vi "XY Scanning with Alazar.vi"() -> ()   [LabVIEW 2018]
uses:
  General/Controls/System Parameters.ctl
  General/Controls/Optical Parameters.ctl
  General/Controls/Vibratome Parameters.ctl
  General/Controls/Translation Stage Parameters.ctl
  Hardware Mfg/Thorlabs Translation Stages/Controls/Translation Stage Cluster.ctl
  General/Controls/Translation Stage Types.ctl
  General/Controls/Imaging Parameters.ctl
  General/Controls/Scan Direction.ctl
  Hardware Mfg/AlazarTech SDK/Controls/Clock Controls.ctl
  Hardware Mfg/AlazarTech SDK/Controls/Alazar Device ID.ctl
  Hardware Mfg/AlazarTech SDK/Controls/Channel Input Controls.ctl
  Hardware Mfg/AlazarTech SDK/Controls/General Trigger Settings.ctl
  Hardware Mfg/AlazarTech SDK/Controls/Trigger Engine Controls.ctl
  Hardware Mfg/AlazarTech SDK/Controls/Alazar Acquisition Settings.ctl
  Hardware Mfg/AlazarTech SDK/Controls/Alazar Engine Actions.ctl
  <vilib>/ErrorRing/Error Ring.xnode
panel:
  out "error out":errorcluster
  in  "stop":bool
  in  "Acq Settings":T1={"Window Type"=1, "Record Length"=1536, "Footer"=0, "Output Format"=11, "Offset"=0, "Records Per Buffer"=1000, "Records Count (Records/Acq)"=2147483647} {"Window Type" items=["DSP_WINDOW_NONE", "DSP_WINDOW_HANNING", "DSP_WINDOW_HAMMING", "DSP_WINDOW_BLACKMAN", "DSP_WINDOW_BLACKMAN_HARRIS", "DSP_WINDOW_BARTLETT"]; "Footer" items=["FOOTER_NONE", "FOOTER_NPT"]; "Output Format" items=["FLOAT_AMP2"=10, "FLOAT_LOG"=11]}
  in  "Trigger Settings":T4={"General Trigger Settings"={"Trigger Operation"=0, "Coupling ID"=2, "Range ID"=0, "Delay"=0, "Timeout Ticks"=0, "Mode"=0, "Parameter"=0}, "Trigger Engine 1"={"Trigger Engine"=0, "Source"=0, "Slope"=1, "Level"=0}, "Trigger Engine 2"={"Trigger Engine"=0, "Source"=0, "Slope"=1, "Level"=0}} {"General Trigger Settings"."Trigger Operation" items=["J", "K", "J OR K", "J AND K", "J XOR K", "J AND NOT K", "NOT J AND K"]; "General Trigger Settings"."Coupling ID" items=["AC"=1, "DC"=2]; "General Trigger Settings"."Range ID" items=["5 V", "1 V", "TTL"]; "Trigger Engine 1"."Trigger Engine" items=["J", "K"]; "Trigger Engine 1"."Source" items=["A", "B", "External", "Disable", "C", "D"]; "Trigger Engine 1"."Slope" items=["Positive"=1, "Negative"=2]; "Trigger Engine 2"."Trigger Engine" items=["J", "K"]; "Trigger Engine 2"."Source" items=["A", "B", "External", "Disable", "C", "D"]; "Trigger Engine 2"."Slope" items=["Positive"=1, "Negative"=2]}
  in  "Ch B Input Control":T5={"Channel"=1, "Coupling"=2, "Range"=10, "Impedance"=2} {"Channel" items=["A"=1, "B"=2, "C"=4, "D"=8]; "Coupling" items=["AC"=1, "DC"=2]; "Range" items=["20 mV"=1, "40 mV"=2, "50 mV"=3, "80 mV"=4, "100 mV"=5, "200 mV"=6, "400 mV"=7, "500 mV"=8, "800 mV"=9, "1 V"=10, "1.25 V"=33, "2 V"=11, "4 V"=12, "5 V"=13, "8 V"=14, "10 V"=15, "20 V"=16]; "Impedance" items=["1 MOhm"=1, "50 Ohm"=2, ""=0]}
  in  "Ch A Input Control":T5={"Channel"=1, "Coupling"=2, "Range"=10, "Impedance"=2} {"Channel" items=["A"=1, "B"=2, "C"=4, "D"=8]; "Coupling" items=["AC"=1, "DC"=2]; "Range" items=["20 mV"=1, "40 mV"=2, "50 mV"=3, "80 mV"=4, "100 mV"=5, "200 mV"=6, "400 mV"=7, "500 mV"=8, "800 mV"=9, "1 V"=10, "1.25 V"=33, "2 V"=11, "4 V"=12, "5 V"=13, "8 V"=14, "10 V"=15, "20 V"=16]; "Impedance" items=["1 MOhm"=1, "50 Ohm"=2, ""=0]}
  in  "Device ID":T6={"System ID"=1, "Board ID"=1}
  in  "Capture Clock":T7={"Source"=1, "Sample Rate"=30, "Edge"=0, "Decimation"=0}
  in  "System Parameters":T8={"Optical Parameters"={"Obj. Focal Length [mm]"=45.0, "Scan Lens EFL[mm]"=60.0, "Tube Lens EFL[mm]"=180.0, "Galvo V Range (+/-)"=10.0, "Galvo Max Half Angle [Deg]"=19.0, "Max Galvo Range[%]"=0.0}, "Vibratome"={"Z Bottom [mm]"=0.0, "Pre Cut Dwell [s]"=0.0, "Blade Frequency [RPM]"=0, "Slice Speed [mm/s]"=0.0, "Post Cut Dwell [s]"=0.0, "Ramp Time [s]"=0.0, "Start X [mm]"=0.0, "Start Y [mm]"=0.0, "Slice Length [mm]"=0.0, "Slice Axis"=enum."Y Axis", "Controller VISA Ref"="COM4"}, "Table Stages"={"X Stage"={"Position"=0.0, "Is.Enabled?"=FALSE, "Is.Connected?"=FALSE, "Device SN"="45876539", "AccelerationMaximum"=0.0, "VelocityMaximum"=0.0, "Acceleration"=0.0, "Velocity"=0.0, "waitTimeout (ms)"=0, "Model"=enum."None", "Is.Homed?"=FALSE}, "Y Stage"={"Position"=0.0, "Is.Enabled?"=FALSE, "Is.Connected?"=FALSE, "Device SN"="45876539", "AccelerationMaximum"=0.0, "VelocityMaximum"=0.0, "Acceleration"=0.0, "Velocity"=0.0, "waitTimeout (ms)"=0, "Model"=enum."None", "Is.Homed?"=FALSE}, "Z Stage"={"Position"=0.0, "Is.Enabled?"=FALSE, "Is.Connected?"=FALSE, "Device SN"="45876539", "AccelerationMaximum"=0.0, "VelocityMaximum"=0.0, "Acceleration"=0.0, "Velocity"=0.0, "waitTimeout (ms)"=0, "Model"=enum."None", "Is.Homed?"=FALSE}}, "Imaging Parameter"={"Raster Scan Direction"=enum."Uni Directional", "Pixel Dwell Time [Clock Cycles]"=1, "Flyback Time [Clock Cycles]"=10, "XY Center [um]"={"X"=1.0, "Y"=1.0}, "Pixel Step Size [um]"=50.0, "XY Image Size"=enum."256 x 256", "Custom"=TRUE, "Custom Size"={"X"=10, "Y"=10}, "Line Averages"=1}} {"Imaging Parameter"."Line Averages" min=1 max=30 step=1; "Imaging Parameter"."Flyback Time [Clock Cycles]" max=10 step=1; "Imaging Parameter"."Pixel Step Size [um]" min=0.0 max=10.0 step=0.01; "Imaging Parameter"."Custom Size"."Y" min=1 max=30 step=1; "Imaging Parameter"."Custom Size"."X" min=1 max=30 step=1; "Imaging Parameter"."XY Center [um]"."Y" min=1.0 max=30.0 step=1.0; "Imaging Parameter"."XY Center [um]"."X" min=1.0 max=30.0 step=1.0; "Imaging Parameter"."Pixel Dwell Time [Clock Cycles]" max=10 step=1}
  in  "Galvo HW Parameters":T16={"Analog Out Channel"="Dev1/ao0", "Min Voltage"=-5.0, "Max Voltage"=5.0, "Pixel Clock Source"="OnboardClock", "Sample Rate"=1000.0, "Line Clock Out Ch"=""}
  # "X"
  # "X"
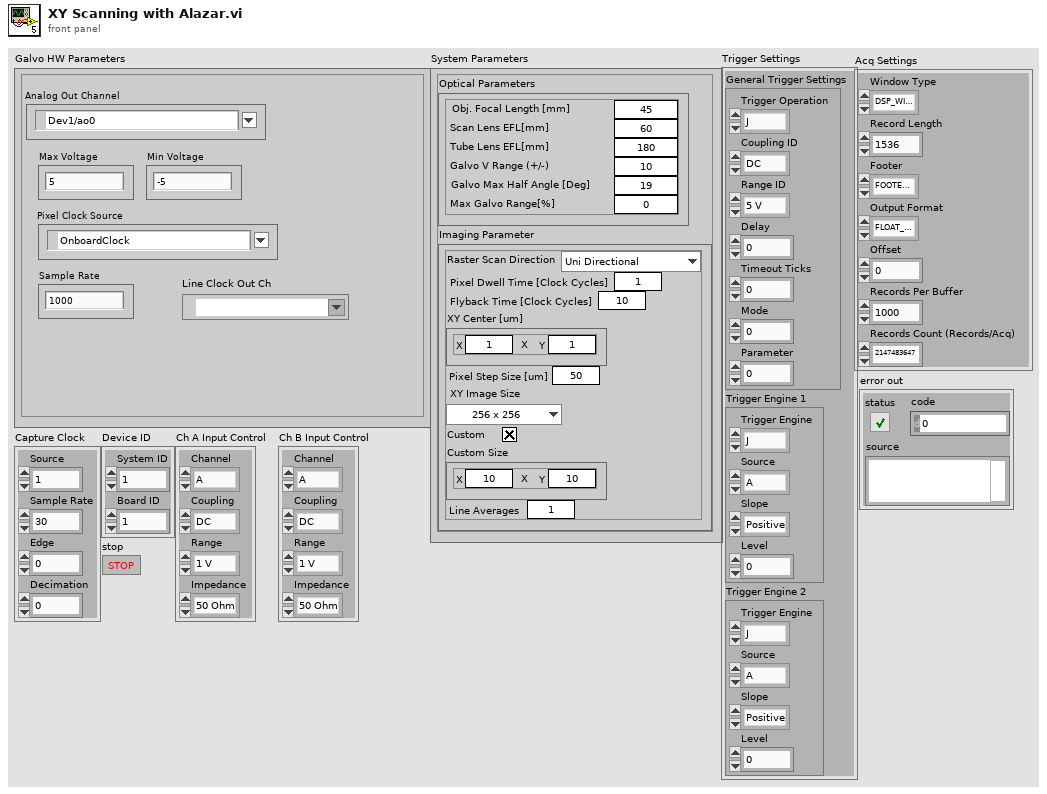
[diagram p1: front panel]
types:
  T1 = typedef "Alazar Acquisition Settings.ctl" = cluster{"Window Type":u32, "Record Length":u32, "Footer":u32, "Output Format":u32, "Offset":u32, "Records Per Buffer":u32, "Records Count (Records/Acq)":u32}
  T2 = typedef "General Trigger Settings.ctl" = cluster{"Trigger Operation":u32, "Coupling ID":u32, "Range ID":u32, "Delay":u32, "Timeout Ticks":u32, "Mode":u32, "Parameter":u32}
  T3 = typedef "Trigger Engine Controls.ctl" = cluster{"Trigger Engine":u32, "Source":u32, "Slope":u32, "Level":u32}
  T4 = cluster{"General Trigger Settings":T2, "Trigger Engine 1":T3, "Trigger Engine 2":T3}
  T5 = typedef "Channel Input Controls.ctl" = cluster{"Channel":u8, "Coupling":u32, "Range":u32, "Impedance":u32}
  T6 = typedef "Alazar Device ID.ctl" = cluster{"System ID":u32, "Board ID":u32}
  T7 = typedef "Clock Controls.ctl" = cluster{"Source":u32, "Sample Rate":u32, "Edge":u32, "Decimation":u32}
  T8 = typedef "System Parameters.ctl" = cluster{"Optical Parameters":T9, "Vibratome":T10, "Table Stages":T11, "Imaging Parameter":T14}
  T9 = typedef "Optical Parameters.ctl" = cluster{"Obj. Focal Length [mm]":dbl, "Scan Lens EFL[mm]":dbl, "Tube Lens EFL[mm]":dbl, "Galvo V Range (+/-)":dbl, "Galvo Max Half Angle [Deg]":dbl, "Max Galvo Range[%]":dbl}
  T10 = typedef "Vibratome Parameters.ctl" = cluster{"Z Bottom [mm]":dbl, "Pre Cut Dwell [s]":dbl, "Blade Frequency [RPM]":u16, "Slice Speed [mm/s]":dbl, "Post Cut Dwell [s]":dbl, "Ramp Time [s]":dbl, "Start X [mm]":dbl, "Start Y [mm]":dbl, "Slice Length [mm]":dbl, "Slice Axis":enum16{"X Axis", "Y Axis", "Z Axis"}, "Controller VISA Ref":refnum<visa-resource-name>}
  T11 = typedef "Translation Stage Parameters.ctl" = cluster{"X Stage":T12, "Y Stage":T12, "Z Stage":T12}
  T12 = typedef "Translation Stage Cluster.ctl" = cluster{"Position":dbl, "Is.Enabled?":bool, "Is.Connected?":bool, "Device SN":string, "AccelerationMaximum":dbl, "VelocityMaximum":dbl, "Acceleration":dbl, "Velocity":dbl, "waitTimeout (ms)":i32, "Model":T13, "Is.Homed?":bool}
  T13 = typedef "Translation Stage Types.ctl" = enum16{"None", "Thorlabs LTS", "Thorlabs MLJ"}
  T14 = typedef "Imaging Parameters.ctl" = cluster{"Raster Scan Direction":T15, "Pixel Dwell Time [Clock Cycles]":u16, "Flyback Time [Clock Cycles]":u16, "XY Center [um]":cluster{"X":dbl, "Y":dbl}, "Pixel Step Size [um]":dbl, "XY Image Size":enum16{"32 x 32", "64 x 64", "128 x 128", "256 x 256", "512 x 512", "1024 x 1024", "2048 x 2048"}, "Custom":bool, "Custom Size":cluster{"X":u16, "Y":u16}, "Line Averages":u8}
  T15 = typedef "Scan Direction.ctl" = enum16{"Uni Directional", "Bi Directional", "None"}
  T16 = cluster{"Analog Out Channel":tag, "Min Voltage":dbl, "Max Voltage":dbl, "Pixel Clock Source":tag, "Sample Rate":dbl, "Line Clock Out Ch":tag}
  T17 = typedef "Alazar Engine Actions.ctl" = enum16{"Init", "Config Clock", "Config Ch", "Config Trig", "Config Acq.", "Acquire", "UnInit"}
  T18 = enum16{"Init", "Calc & Write Scan Pattern", "Start Galvo Task", "Is Task Done?", "Stop Galvo", "Uninit"}
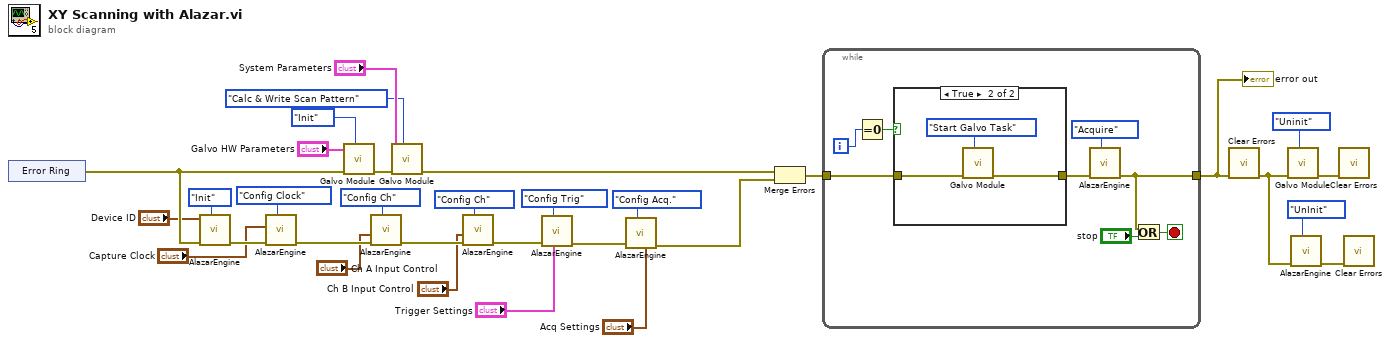
[diagram p0: block diagram]
diagram:
  n1 = xnode "Error Ring"() -> ("error out"=w23:errorcluster)
  n2 = call "AlazarEngine.vi"("Action"=Alazar_Engine_Actions."Init", "error in (no error)"=w23, "Device ID"="Device ID") -> ("error out"=w26:errorcluster)  [unwired: 7 in, 1 out]
  n3 = call "AlazarEngine.vi"("Action"=Alazar_Engine_Actions."Config Clock", "error in (no error)"=w26, "Capture Clock"="Capture Clock") -> ("error out"=w25:errorcluster)  [unwired: 7 in, 1 out]
  n4 = call "Galvo Module.vi"("Action"=T18."Init", "error in (no error)"=w23, "Galvo HW Parameters"="Galvo HW Parameters") -> ("error out"=w30:errorcluster)  [unwired: 7 in, 1 out]
  n5 = call "AlazarEngine.vi"("Action"=Alazar_Engine_Actions."Config Ch", "error in (no error)"=w25, "Ch Input Control"="Ch A Input Control") -> ("error out"=w24:errorcluster)  [unwired: 7 in, 1 out]
  n6 = call "Galvo Module.vi"("Action"=T18."Calc & Write Scan Pattern", "error in (no error)"=w30, "System Parameters"="System Parameters") -> ("error out"=w29:errorcluster)  [unwired: 7 in, 1 out]
  n7 = call "AlazarEngine.vi"("Action"=Alazar_Engine_Actions."Config Ch", "error in (no error)"=w24, "Ch Input Control"="Ch B Input Control") -> ("error out"=w14:errorcluster)  [unwired: 7 in, 1 out]
  n8 = call "AlazarEngine.vi"("Trigger Settings"="Trigger Settings", "Action"=Alazar_Engine_Actions."Config Trig", "error in (no error)"=w14) -> ("error out"=w11:errorcluster)  [unwired: 7 in, 1 out]
  n9 = call "AlazarEngine.vi"("Acq Settings"="Acq Settings", "Action"=Alazar_Engine_Actions."Config Acq.", "error in (no error)"=w11) -> ("error out"=w7:errorcluster)  [unwired: 7 in, 1 out]
  n10 = Merge Errors(w29, w7) -> (w8:errorcluster)
  n11 = while {
    tunnel: w8 -> [w40]
    tunnel: [w33] -> w6
    i -> [w39]
    stop <- w34 stop-if-true
    n12 = Equal To 0?(x=w39) -> (x = 0?=w38:bool)
    n13 = case shown="True" w38 {
      tunnel: w40 -> [w41 w44]
      tunnel: [w41 w42] -> w37
      frame False {
      }
      frame True {
        n14 = call "Galvo Module.vi"("Action"=T18."Start Galvo Task", "error in (no error)"=w44) -> ("error out"=w42:errorcluster)  [unwired: 8 in, 1 out]
      }
    }
    n15 = call "AlazarEngine.vi"("Action"=Alazar_Engine_Actions."Acquire", "error in (no error)"=w37) -> ("error out"=w33:errorcluster)  [unwired: 8 in, 1 out]
    n16 = Or(x=w33, y="stop") -> (x .or. y?=w34:bool)
  }
  "error out" <- w6
  n17 = call <vilib>:"Clear Errors.vi"("error in (no error)"=w6) -> ("error out"=w3:errorcluster)  [unwired: 5 in, 1 out]
  n18 = call "Galvo Module.vi"("Action"=T18."Uninit", "error in (no error)"=w3) -> ("error out"=w2:errorcluster)  [unwired: 8 in, 1 out]
  n19 = call "AlazarEngine.vi"("Action"=Alazar_Engine_Actions."UnInit", "error in (no error)"=w3) -> ("error out"=w1:errorcluster)  [unwired: 8 in, 1 out]
  n20 = call <vilib>:"Clear Errors.vi"("error in (no error)"=w2) -> ()  [unwired: 5 in, 2 out]
  n21 = call <vilib>:"Clear Errors.vi"("error in (no error)"=w1) -> ()  [unwired: 5 in, 2 out]
